vi "thermocouple.vi"(8 "error in":errorcluster, 9 "max volume":dbl, 10 "volume rise per 1C":dbl, 11 "physical channels":tag="cDAQ4Mod2/ai0") -> (0 "error out":errorcluster, 3 "volume":dbl)   [LabVIEW 2022 SP3]
uses:
  <vilib>/DAQmx/read.llb/DAQmx Read (Analog DBL 1Chan 1Samp).vi
  <vilib>/DAQmx/create/channels.llb/DAQmx Create Channel (AI-Temperature-Thermocouple).vi
  <vilib>/DAQmx/miscellaneous.llb/DAQmx Fill In Error Info.vi
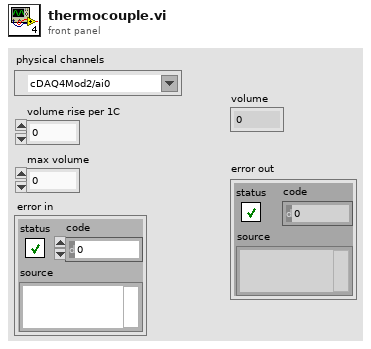
[diagram p1: front panel]
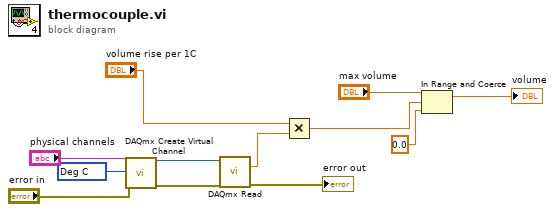
[diagram p0: block diagram]
diagram:
  w3 = 10143 items=["Deg C"=10143, "Deg F"=10144, "Kelvins"=10325, "Deg R"=10145, "From Custom Scale"=10065] ("units")
  n1 = call-poly <vilib>:"DAQmx Create Virtual Channel.vi"("physical channels"="physical channels", "units"=w3, "error in"="error in") -> ("task out"=w12:refnum<k21>, "error out"=w11:errorcluster)  [unwired: 11 in]
  n2 = call-poly <vilib>:"DAQmx Read.vi"("task/channels in"=w12, "error in"=w11) -> ("data"=w9:dbl, "error out"=→"error out":errorcluster)  [unwired: 11 in, 1 out]
  n3 = Multiply(x="volume rise per 1C", y=w9) -> (x*y=w6:dbl)
  n4 = In Range and Coerce(upper limit="max volume", x=w6, lower limit=0.0) -> (coerced(x)=→"volume":dbl)  [unwired: 1 out]
